vi "Get TDMS folder name.vi"(11 "Imaging Protocol":T1) -> (3 "TDMS files folder name":string)   [LabVIEW 2013]
uses:
  Typedefs/Imaging Protocols enum.ctl
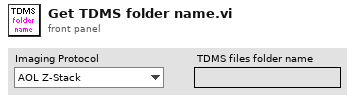
[diagram p1: front panel]
types:
  T1 = typedef "Imaging Protocols enum.ctl" = enum16{"AOL Z-Stack", "Motor Z Stack", "Functional Acquisition", "Single Plane Acquisition", "Volume Acquisition", "Live Imaging", "Live Plane Imaging", "Live Volume Imaging"}
  T2 = typedef "Fixed strings.ctl" = cluster{"ROI file name":string, "Normalised ROI file name":string, "Zplane Pockels values file name":string, "Functional data folder name":string, "Experiment Header file name":string, "Z-stack images folder name":string, "Groups setup rel. path":string, "Groups text file rel. path":string, "TDMS files folder name (F.img)":string, "TDMS files folder name (V.acq)":string, "TDMS files folder name (Pl.acq)":string, "Cycle rel times sequence file":string, "Dynamically called VIs folder name":string, "Time Series folder base name":string}
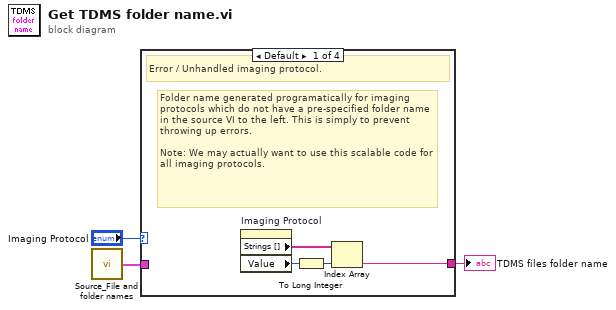
[diagram p0: block diagram]
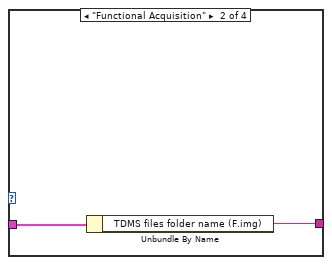
[diagram p2: hidden frame]
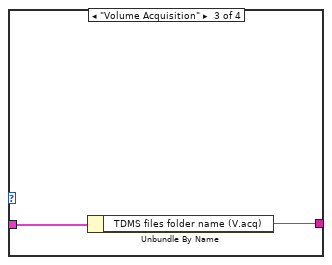
[diagram p3: hidden frame]
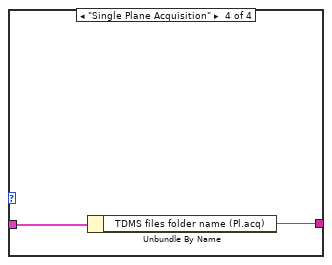
[diagram p4: hidden frame]
diagram:
  n1 = call "Source_File and folder names.vi"() -> ("Fixed strings"=w1:T2)  [unwired: 1 in]
  n2 = case shown="Default" "Imaging Protocol" {
    tunnel: w1 -> [_ w9 w11 w13]
    tunnel: [w4 w8 w10 w12] -> w2
    frame Default {
      # "Folder name generated programatically for imaging\nprotocols which do not have a pre-specified folder name in the source VI to the left. This is simply to prevent throwing up errors.\n\nNote: We may actually want to use this scalable code for all imaging protocols."
      # "Error / Unhandled imaging protocol."
      n3 = property on="Imaging Protocol" class="Enum (strict)"() -> ("Strings []"=w7:string[], "Value"=w6:T1)  [unwired: 2 in, 2 out]
      n4 = To Long Integer(number=w6) -> (32bit integer=w5:i32)
      n5 = Index Array(array=w7, index=w5) -> (element=w4:string)
    }
    frame "Functional Acquisition" {
      n6 = Unbundle By Name(w9) -> ("TDMS files folder name (F.img)"=w8:string)
    }
    frame "Volume Acquisition" {
      n7 = Unbundle By Name(w11) -> ("TDMS files folder name (V.acq)"=w10:string)
    }
    frame "Single Plane Acquisition" {
      n8 = Unbundle By Name(w13) -> ("TDMS files folder name (Pl.acq)"=w12:string)
    }
  }
  "TDMS files folder name" <- w2
